vi "Init Dll.vi"(8 "error in (no error)":errorcluster, 10 "en_hard_watchdog":u32, 11 "en_log":u32) -> (0 "error out":errorcluster, 3 "function return":i32)   [LabVIEW 2021, in "vmmso.lvlib"]
doc: "DLL_API int WINAPI InitDll(unsigned int en_log, unsigned int en_hard_watchdog);"
uses:
  vmmso.lvlib
  vmmso.dll
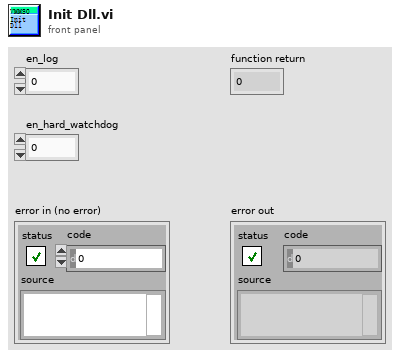
[diagram p1: front panel]
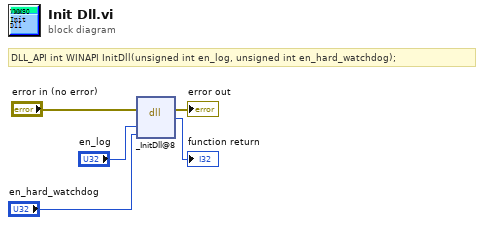
[diagram p0: block diagram]
diagram:
  # "DLL_API int WINAPI InitDll(unsigned int en_log, unsigned int en_hard_watchdog);"
  n1 = dll-call lib="O:/MSO/library/demo-Labview/vmmso/vmmso.*" fn="_InitDll@8"(error in="error in (no error)", "en_log"="en_log", "en_hard_watchdog"="en_hard_watchdog") -> (error out=→"error out":errorcluster, →"function return":i32)  [unwired: 4 in, 1 out]
